vi "SPC_stream_start_condition.vi"(5 "Start OR Mask":u32 format="%x", 6 "Stream Handle":i16, 7 "Start AND Mask":u32 format="%x", 8 "Error In":errorcluster, 9 "Start Time":dbl, 11 "DLL Path":path) -> (0 "Error Out":errorcluster, 3 "DLL Path":path, 4 "Stream Handle":i16)   [LabVIEW 2017]
doc: "-start_time: macro time (in sec) at which extracting photons will start ( during call to SPC_get_photons_from_stream)\n-start_OR_mask: bitwise OR mask used to define start of extracting photons from the stream ( in addition to 'start_time'), bits 31-28 - markers M3-M0, bits 27-0 - routing channels 27-0 \n-start_AND_mask: bitwise AND mask used to define start of extracting photons from the stream ( in addition to 'start_time'), bits 31-28 - markers M3-M0, bits 27-0 - routing channels 27-0 \n\nThe procedure is used to define start of extracting photons from buffered stream 'stream_hndl' during SPC_get_photons_from_stream call. \nStart_time and OR/AND masks can be used all together.\nAll photons (markers) are ignored until the macro time in the stream reaches 'start_time' \nvalue. From this moment appearance of specified markers/channels is tested according to start_OR(AND)_mask. \nStart condition is found when minimum one of markers/channels defined in start_OR_mask appears in the stream (since 'start_time').\nStart condition is also found when all of markers/channels defined in start_AND_mask\nappeared in the stream (since 'start_time').\nSPC_get_photons_from_stream returns an error, when start condition cannot be found in the stream. \nWhile extracting photons during running measurement, start condition (if defined) can be found later after reading new portion of photons data from FIFO to the stream (using SPC_read_fifo_to_stream).\n\ninfo@becker-hickl.com"
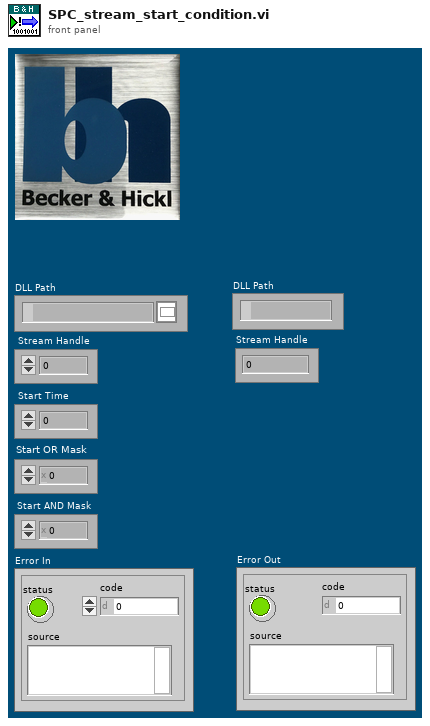
[diagram p1: front panel]
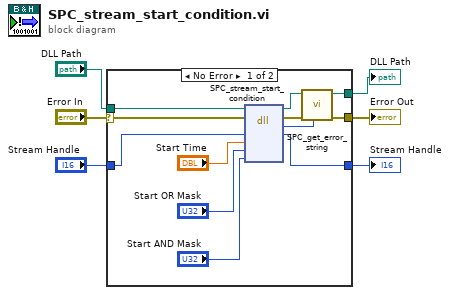
[diagram p0: block diagram]
diagram:
  n1 = case shown="No Error" "Error In" {
    selector: "Error In" -> [w14 w20]
    tunnel: "DLL Path" -> [w15 w21]
    tunnel: [w12 w20] -> w4
    tunnel: [w9 w21] -> w3
    tunnel: "Stream Handle" -> [w8 w19]
    tunnel: [w7 w19] -> w1
    frame No Error {
      n2 = dll-call lib="D:/spcm/lib/lab_view/lv10.0/spcm32.dll" fn="SPC_stream_start_condition"(path in=w15, error in=w14, "stream_hndl"=w8, "start_time"="Start Time", "start_OR_mask"="Start OR Mask", "start_AND_mask"="Start AND Mask") -> (path out=w10:path, error out=w13:errorcluster, "return type"=w11:i16, "stream_hndl"=w7:i16)  [unwired: 4 in]
      n3 = call "SPC_get_error_string.vi"("ErrorID"=w11, "Error In"=w13, "DLL Path"=w10) -> ("Error Out"=w12:errorcluster, "DLL Path"=w9:path)  [unwired: 6 in, 1 out]
    }
    frame Error {
    }
  }
  "Error Out" <- w4
  "DLL Path" <- w3
  "Stream Handle" <- w1
